vi "OE1201_Query PLL&Overload.vi"(8 "Error in (no error)":errorcluster caption="error out（no error）", 9 "Remote Mode":u16(ring) items=["USB", "RS232"], 11 "VISA resource name":refnum<visa-resource-name>) -> (0 "Error out":errorcluster caption="error out", 1 "Output String":string, 2 "OE1201_Query PLL&Overload":T1, 3 "VISA resource  out":refnum<visa-resource-name>)   [LabVIEW 2011]
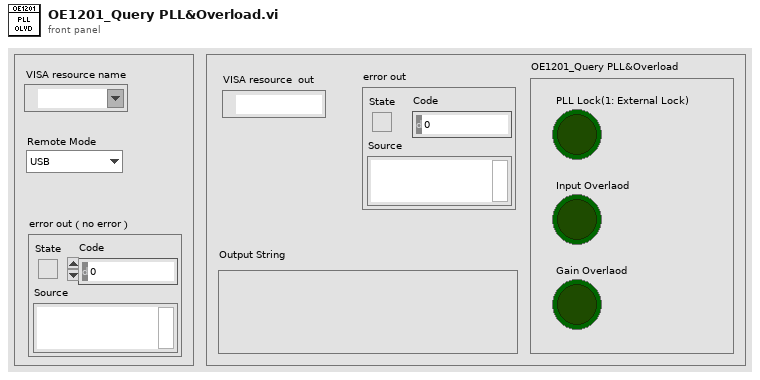
[diagram p1: front panel]
types:
  T1 = cluster{"Input Overlaod":bool, "Gain Overlaod":bool, "PLL Lock(1: External Lock)":bool}
  T2 = enum16{"ISRC", "IGND", "ICPL", "ILIN", "PHAS", "FMOD", "RSLP", "FREQ", "SWPT", "SLLM", "SULM", "SSLL", "SSLG", "STLM", "SWRM", "IRNG", "SENS", "RMOD", "OFLT", "OFSL", "SYNC", "DMOD", "HARM", "DARB", "SWVT", "SLVL", "SVLL", "SVUL", "SVSL", "SVSG", "SVTM", "SVRM", "RALL", "SNAP", "OUTP", "OAUX", "COUT", "CAUX", "COFP", "CEXP", "FPOP", "OEXP", "*IDN", "*RST", "OVLD", "INOV", "GNOV", "*PLL", "SSET", "RSET", "AGAN", "APHS", "ARSV", "ASCL", "EQCD", "EQCS", "SPED", "SRAT", "SLEN", "SSLE", "STRG", "SPRM", "STRD", "PAUS", "REST", "SPTS", "TRCA", "TEMP", "RSTU", "IHNZ", "DEQU", "SADD", "ARNG", "CSPE", "ISRCD", "IGNDD", "ICPLD", "ILIND", "PHASD", "FMODD", "RSLPD", "FREQD", "SWPTD", "SLLMD", "SULMD", "SSLLD", "SSLGD", "STLMD", "SWRMD", "SENSD", "RMODD", "OFLTD", "OFSLD", "SYNCD", "HARMD", "EQCDD", "EQCSD", "SNAPD", "OUTPD", "SWVTD", "SLVLD", "SVLLD", "SVULD", "SVSLD", "SVSGD", "SVTMD", "SVRMD", "SVDCD", "ARSVD", "AGAND", "APHSD", "ASCLD", "FPOPD", "CAUXD", "OEXPD", "SPEDD", "SRATD", "SLEND", "SSLED", "STRGD", "SPRMD", "STRDD", "PAUSD", "RESTD", "SPTSD", "TRCAD", "*IDND", "*RSTD", "INOVD", "GNOVD", "*PLLD", "SSETD", "RSETD"}
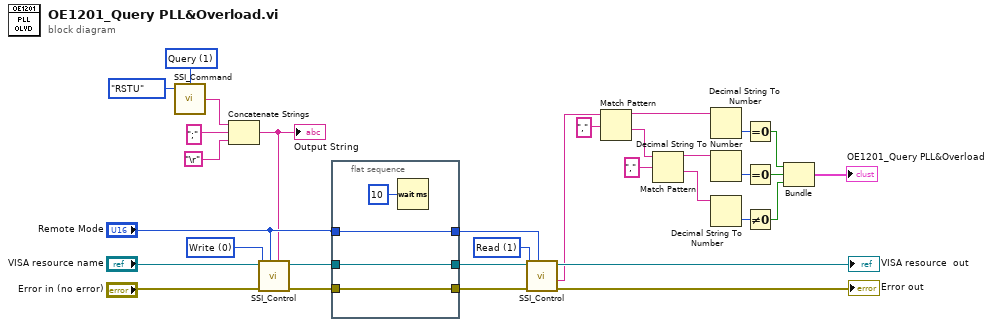
[diagram p0: block diagram]
diagram:
  w19 = u16 1 items=["Write", "Read"] ("Control")
  w16 = u16 1 items=["Set", "Query"] ("Opera")
  w31 = u16 0 items=["Write", "Read"] ("Control")
  n1 = call "SSI_Command.vi"("Opera"=w16, "Command Type"=T2."RSTU") -> ("Output string"=w11:string)  [unwired: 2 in]
  n2 = Concatenate Strings(w11, ";", "\r") -> (w20:string)
  "Output String" <- w20
  n3 = call "SSI_Control.vi"("Write Buffer"=w20, "Remote Mode"="Remote Mode", "Error in (no error)"="Error in (no error)", "Control"=w31, "VISA resource name"="VISA resource name") -> ("Error out"=w29:errorcluster, "VISA resource  out"=w28:refnum<visa-resource-name>)  [unwired: 3 in, 2 out]
  n4 = flat-sequence {
    tunnel: [w36] -> w27
    tunnel: w29 -> [w36]
    tunnel: [w35] -> w26
    tunnel: w28 -> [w35]
    tunnel: "Remote Mode" -> [w33]
    tunnel: [w33] -> w25
    frame #0 {
      n5 = Wait (ms)(milliseconds to wait=u32 10 ("等待时间（毫秒）")) -> ()  [unwired: 1 out]
    }
  }
  n6 = call "SSI_Control.vi"("Remote Mode"=w25, "Error in (no error)"=w27, "Control"=w19, "VISA resource name"=w26) -> ("Error out"=→"Error out":errorcluster, "Read Buffer"=w10:string, "VISA resource  out"=→"VISA resource  out":refnum<visa-resource-name>)  [unwired: 4 in, 1 out]
  n7 = Match Pattern(string=w10, regular expression="," ("正则表达式")) -> (before substring=w8:string, after substring=w6:string)  [unwired: 1 in, 2 out]
  n8 = Match Pattern(string=w6, regular expression="," ("正则表达式")) -> (before substring=w5:string, after substring=w4:string)  [unwired: 1 in, 2 out]
  n9 = Decimal String To Number(string=w8) -> (number=w1:i32)  [unwired: 2 in, 1 out]
  n10 = Decimal String To Number(string=w5) -> (number=w2:i32)  [unwired: 2 in, 1 out]
  n11 = Decimal String To Number(string=w4) -> (number=w3:i32)  [unwired: 2 in, 1 out]
  n12 = Equal To 0?(x=w1) -> (x = 0?=w18:bool)
  n13 = Equal To 0?(x=w2) -> (x = 0?=w21:bool)
  n14 = Not Equal To 0?(x=w3) -> (x != 0?=w15:bool)
  n15 = Bundle(w18, w21, w15) -> (→"OE1201_Query PLL&Overload":cluster{bool, bool, bool})  [unwired: 1 in]
